vi "classes.vi"(0 "HGF_IMAQFactory":refnum<class "HGF_IMAQFactory.lvclass">, 1 "className":string, 5 "error in (no error)":errorcluster) -> (14 "dup HGF_IMAQFactory":refnum<class "HGF_IMAQFactory.lvclass">, 16 "Object":refnum<class>, 19 "error out":errorcluster)   [LabVIEW 2014, in "HGF_IMAQ.lvlib" / "HGF_IMAQFactory.lvclass"]
doc: "This dynamaic dispatch VI contains constant objects of all classes that can be produced by HGF_Factory.\nClass has to be defined by name. \n\nOptionally, you can also specifiy a Class Path String instead, but you have to make sure that all dependencies are available.\n\nChild classes have to override it to define additional classes."
uses:
  HGF_IMAQFactory.lvclass
  HGF_ImaqFg/HGF_ImaqFg.lvclass
  HGF_ImaqDx/HGF_ImaqDx.lvclass
  HGF_DeviceBaseClasses/HGF_DeviceBaseFactory/HGF_DeviceBaseFactory.lvclass
  HGF_Basler_A602f/HGF_Basler_A602f.lvclass
  HGF_Prosilica_GC655/HGF_Prosilica_GC655.lvclass
  HGF_AVT_F033B/HGF_AVT_F033B.lvclass
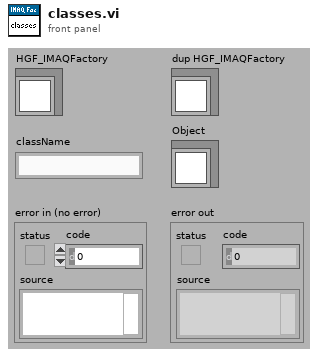
[diagram p1: front panel]
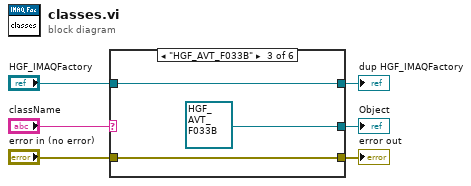
[diagram p0: block diagram]
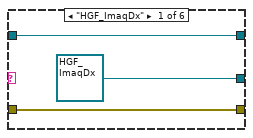
[diagram p2: hidden frame]
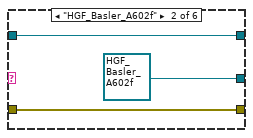
[diagram p3: hidden frame]
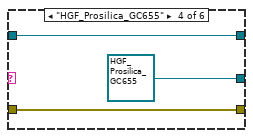
[diagram p4: hidden frame]
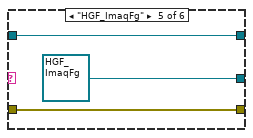
[diagram p5: hidden frame]
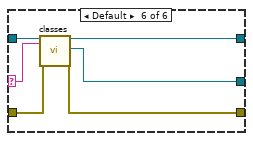
[diagram p6: hidden frame]
diagram:
  n1 = case shown="\"HGF_AVT_F033B\"" "className" {
    selector: "className" -> [_ _ _ _ _ w22]
    tunnel: "HGF_IMAQFactory" -> [w9 w12 w15 w18 w21 w27]
    tunnel: "error in (no error)" -> [w8 w10 w14 w17 w20 w26]
    tunnel: [w9 w12 w15 w18 w21 w25] -> w3
    tunnel: [refnum<class "HGF_ImaqDx.lvclass"> refnum ("HGF_IMAQ.lvlib:HGF_ImaqDx.lvclass") refnum<class "HGF_Basler_A602f.lvclass"> refnum ("HGF_IMAQ.lvlib:HGF_Basler_A602f.lvclass") refnum<class "HGF_AVT_F033B.lvclass"> refnum ("HGF_IMAQ.lvlib:HGF_AVT_F033B.lvclass") refnum<class "HGF_Prosilica_GC655.lvclass"> refnum ("HGF_IMAQ.lvlib:HGF_Prosilica_GC655.lvclass") refnum<class "HGF_ImaqFg.lvclass"> refnum ("HGF_IMAQ.lvlib:HGF_ImaqFg.lvclass") w24] -> w2
    tunnel: [w8 w10 w14 w17 w20 w23] -> w1
    frame "HGF_ImaqDx" {
    }
    frame "HGF_Basler_A602f" {
    }
    frame "HGF_AVT_F033B" {
    }
    frame "HGF_Prosilica_GC655" {
    }
    frame "HGF_ImaqFg" {
    }
    frame Default {
      n2 = call-parent "classes.vi"("HGF_Factory"=w27, "className"=w22, "error in (no error)"=w26) -> ("HGF_Factory dup"=w25:refnum<class "HGF_IMAQFactory.lvclass">, "Object"=w24:refnum<class>, "error out"=w23:errorcluster)  [unwired: 14 out]
    }
  }
  "error out" <- w1
  "dup HGF_IMAQFactory" <- w3
  "Object" <- w2
